vi "instr.UT61E.vi"(2 "error in (no error)":errorcluster caption="错误输入（无错误）", 3 "串口开关":bool, 4 "档位选择":enum16{"电流/mA", "电流/A", "电压/V"}(ring), 5 "VISA resource name":refnum<visa-resource-name> caption="VISA资源名称") -> (0 "error out":errorcluster caption="错误输出", 1 "结果":dbl)   [LabVIEW 2012, in "Lib_UEL.ATE.lvlib" / "Lib_Instrument.lvlib"]
uses:
  Lib_Instrument.lvlib
  <vilib>/Instr/_visa.llb/VISA Configure Serial Port (Instr).vi
panel:
  out "读取缓冲区":string
  # "1.电流电压均为直流测试时有效，且应打在对应的档位\n2.结果的单位与选择的单位一致\n                                             2013.6.18 Tina"
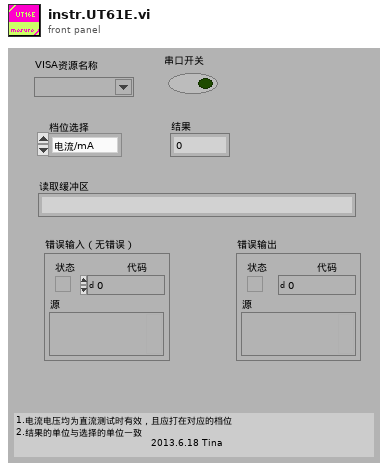
[diagram p1: front panel]
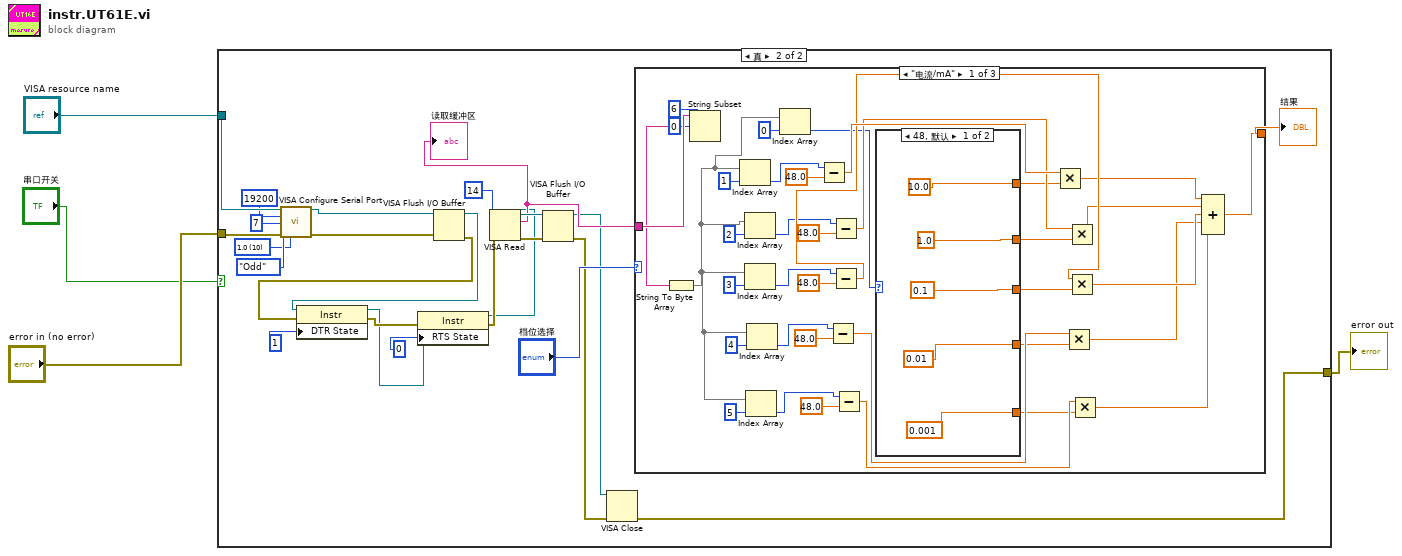
[diagram p0: block diagram]
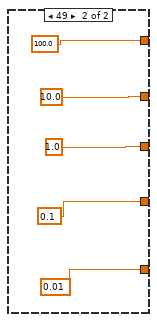
[diagram p3: hidden frame]
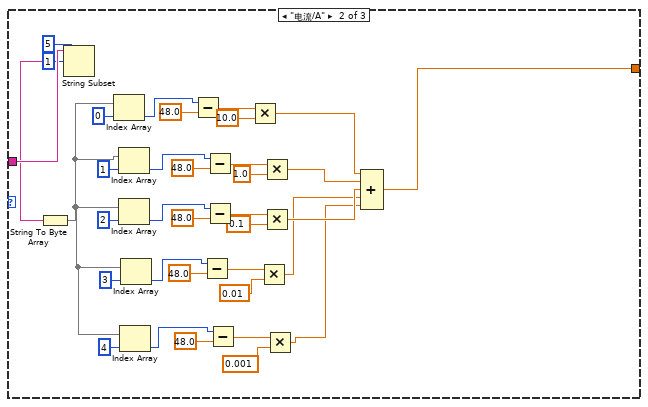
[diagram p4: hidden frame]
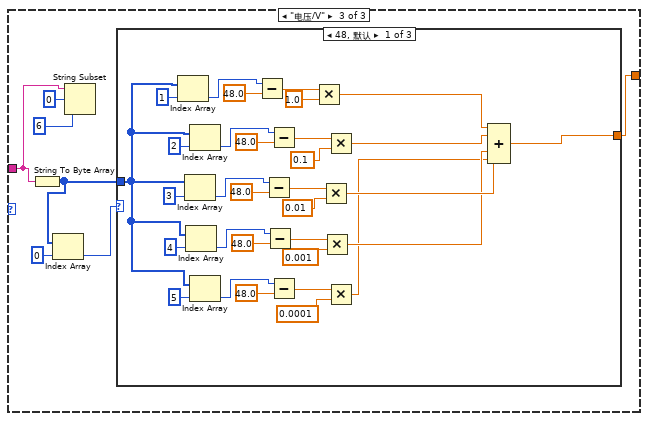
[diagram p5: hidden frame]
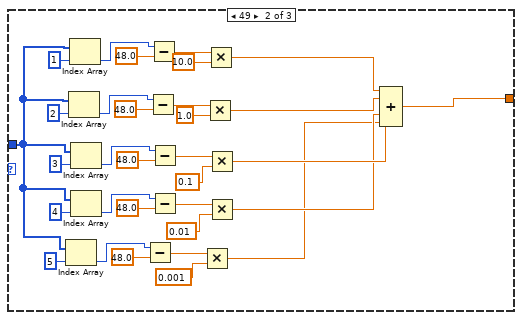
[diagram p6: hidden frame]
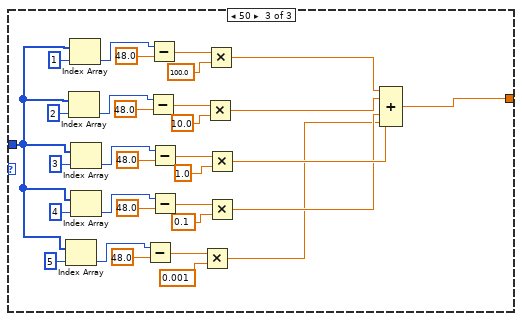
[diagram p7: hidden frame]
diagram:
  n1 = case shown="真" "串口开关" {
    tunnel: "VISA resource name" -> [_ w30]
    tunnel: "error in (no error)" -> [w5 w29]
    tunnel: [w5 w8] -> w1
    frame False {
    }
    frame True {
      w25 = u16 10 items=["1.0"=10, "1.5"=15, "2.0"=20] ("stop bits (10: 1 bit)")
      n2 = call-poly "VISA Configure Serial Port"("VISA resource name"=w30, "baud rate (9600)"=u32 19200, "data bits (8)"=u16 7, "parity (0:none)"=enum16{"None", "Odd", "Even", "Mark", "Space"}."Odd", "error in (no error)"=w29, "stop bits (10: 1 bit)"=w25) -> ("VISA resource name out"=w7:refnum<visa-resource-name>, "error out"=w6:errorcluster)  [unwired: 8 in]
      n3 = VISA Flush I/O Buffer(VISA resource name=w7, error in (no error)=w6) -> (VISA resource name out=w16:refnum<visa-resource-name>, error out=w15:errorcluster)  [unwired: 1 in]
      n4 = property class="Instr"(reference=w16, error in=w15, "DTR State"=1) -> (reference out=w13:refnum<visa-resource-name>, error out=w14:errorcluster)
      n5 = property class="Instr"(reference=w13, error in=w14, "RTS State"=0) -> (reference out=w11:refnum<visa-resource-name>, error out=w12:errorcluster)
      n6 = VISA Read(VISA resource name=w11, byte count=u32 14 ("字节总数"), error in (no error)=w12) -> (VISA resource name out=w23:refnum<visa-resource-name>, read buffer=w21:string, error out=w22:errorcluster)  [unwired: 1 out]
      "读取缓冲区" <- w21
      n7 = VISA Flush I/O Buffer(VISA resource name=w23, error in (no error)=w22) -> (VISA resource name out=w10:refnum<visa-resource-name>, error out=w9:errorcluster)  [unwired: 1 in]
      n8 = VISA Close(VISA resource name=w10, error in (no error)=w9) -> (error out=w8:errorcluster)
      n9 = case shown="\"电流/mA\"" "档位选择" {
        tunnel: w21 -> [w68 w114 w119]
        tunnel: [w34 w79 w115] -> w19
        frame "电流/mA" {
          n10 = String Subset(string=w68, offset (0)=0 ("偏移量(0)"), length (rest)=6 ("长度（剩余）")) -> (substring=w65:string)
          n11 = String To Byte Array(string=w65) -> (unsigned byte array=w32:u8[])
          n12 = Index Array(array=w32, index=1 ("索引")) -> (element=w45:u8)
          n13 = Index Array(array=w32, index=2 ("索引")) -> (element=w46:u8)
          n14 = Index Array(array=w32, index=3 ("索引")) -> (element=w47:u8)
          n15 = Index Array(array=w32, index=5 ("索引")) -> (element=w49:u8)
          n16 = Index Array(array=w32, index=4 ("索引")) -> (element=w48:u8)
          n17 = Index Array(array=w32, index=0 ("索引")) -> (element=w31:u8)
          n18 = Subtract(x=w45, y=48.0) -> (x-y=w58:dbl)
          n19 = Subtract(x=w48, y=48.0) -> (x-y=w52:dbl)
          n20 = Subtract(x=w46, y=48.0) -> (x-y=w57:dbl)
          n21 = Subtract(x=w47, y=48.0) -> (x-y=w55:dbl)
          n22 = Subtract(x=w49, y=48.0) -> (x-y=w51:dbl)
          n23 = case shown="48, 默认" w31 {
            tunnel: [10.0 ("y") 100.0 ("y")] -> w44
            tunnel: [1.0 ("y") 10.0 ("y")] -> w43
            tunnel: [0.1 ("y") 1.0 ("y")] -> w42
            tunnel: [0.01 ("y") 0.1 ("y")] -> w41
            tunnel: [0.001 ("y") 0.01 ("y")] -> w40
            frame 48, Default {
            }
            frame 49 {
            }
          }
          n24 = Multiply(x=w58, y=w44) -> (x*y=w39:dbl)
          n25 = Multiply(x=w52, y=w41) -> (x*y=w36:dbl)
          n26 = Multiply(x=w57, y=w43) -> (x*y=w38:dbl)
          n27 = Multiply(x=w55, y=w42) -> (x*y=w37:dbl)
          n28 = Multiply(x=w51, y=w40) -> (x*y=w35:dbl)
          n29 = Compound Arithmetic op=ADD(w39, w38, w37, w36, w35) -> (w34:dbl)
        }
        frame "电流/A" {
          n30 = String Subset(string=w114, offset (0)=1 ("偏移量(0)"), length (rest)=5 ("长度（剩余）")) -> (substring=w111:string)
          n31 = String To Byte Array(string=w111) -> (unsigned byte array=w110:u8[])
          n32 = Index Array(array=w110, index=0 ("索引")) -> (element=w90:u8)
          n33 = Index Array(array=w110, index=1 ("索引")) -> (element=w91:u8)
          n34 = Index Array(array=w110, index=2 ("索引")) -> (element=w92:u8)
          n35 = Index Array(array=w110, index=4 ("索引")) -> (element=w94:u8)
          n36 = Index Array(array=w110, index=3 ("索引")) -> (element=w93:u8)
          n37 = Subtract(x=w90, y=48.0) -> (x-y=w103:dbl)
          n38 = Subtract(x=w93, y=48.0) -> (x-y=w97:dbl)
          n39 = Subtract(x=w91, y=48.0) -> (x-y=w102:dbl)
          n40 = Subtract(x=w92, y=48.0) -> (x-y=w100:dbl)
          n41 = Subtract(x=w94, y=48.0) -> (x-y=w96:dbl)
          n42 = Multiply(x=w103, y=10.0) -> (x*y=w84:dbl)
          n43 = Multiply(x=w97, y=0.01) -> (x*y=w81:dbl)
          n44 = Multiply(x=w102, y=1.0) -> (x*y=w83:dbl)
          n45 = Multiply(x=w100, y=0.1) -> (x*y=w82:dbl)
          n46 = Multiply(x=w96, y=0.001) -> (x*y=w80:dbl)
          n47 = Compound Arithmetic op=ADD(w84, w83, w82, w81, w80) -> (w79:dbl)
        }
        frame "电压/V" {
          n48 = String To Byte Array(string=w119) -> (unsigned byte array=w116:u8[])
          n49 = Index Array(array=w116, index=0 ("索引")) -> (element=w117:u8)
          n50 = String Subset(string=w119, offset (0)=0 ("偏移量(0)"), length (rest)=6 ("长度（剩余）")) -> ()  [unwired: 1 out]
          n51 = case shown="48, 默认" w117 {
            tunnel: w116 -> [w124 w154 w186]
            tunnel: [w138 w170 w202] -> w115
            frame 48, Default {
              n52 = Index Array(array=w124, index=1 ("索引")) -> (element=w150:u8)
              n53 = Index Array(array=w124, index=3 ("索引")) -> (element=w142:u8)
              n54 = Index Array(array=w124, index=4 ("索引")) -> (element=w133:u8)
              n55 = Index Array(array=w124, index=2 ("索引")) -> (element=w149:u8)
              n56 = Index Array(array=w124, index=5 ("索引")) -> (element=w126:u8)
              n57 = Subtract(x=w150, y=48.0) -> (x-y=w151:dbl)
              n58 = Subtract(x=w142, y=48.0) -> (x-y=w143:dbl)
              n59 = Subtract(x=w133, y=48.0) -> (x-y=w132:dbl)
              n60 = Subtract(x=w149, y=48.0) -> (x-y=w148:dbl)
              n61 = Subtract(x=w126, y=48.0) -> (x-y=w127:dbl)
              n62 = Multiply(x=w151, y=1.0) -> (x*y=w141:dbl)
              n63 = Multiply(x=w143, y=0.01) -> (x*y=w139:dbl)
              n64 = Multiply(x=w132, y=0.001) -> (x*y=w123:dbl)
              n65 = Multiply(x=w148, y=0.1) -> (x*y=w140:dbl)
              n66 = Multiply(x=w127, y=0.0001) -> (x*y=w122:dbl)
              n67 = Compound Arithmetic op=ADD(w141, w140, w139, w123, w122) -> (w138:dbl)
            }
            frame 49 {
              n68 = Index Array(array=w154, index=5 ("索引")) -> (element=w158:u8)
              n69 = Index Array(array=w154, index=2 ("索引")) -> (element=w181:u8)
              n70 = Index Array(array=w154, index=1 ("索引")) -> (element=w182:u8)
              n71 = Index Array(array=w154, index=3 ("索引")) -> (element=w174:u8)
              n72 = Index Array(array=w154, index=4 ("索引")) -> (element=w165:u8)
              n73 = Subtract(x=w158, y=48.0) -> (x-y=w159:dbl)
              n74 = Subtract(x=w181, y=48.0) -> (x-y=w180:dbl)
              n75 = Subtract(x=w182, y=48.0) -> (x-y=w183:dbl)
              n76 = Subtract(x=w174, y=48.0) -> (x-y=w175:dbl)
              n77 = Subtract(x=w165, y=48.0) -> (x-y=w164:dbl)
              n78 = Multiply(x=w159, y=0.001) -> (x*y=w155:dbl)
              n79 = Multiply(x=w180, y=1.0) -> (x*y=w172:dbl)
              n80 = Multiply(x=w183, y=10.0) -> (x*y=w173:dbl)
              n81 = Multiply(x=w175, y=0.1) -> (x*y=w171:dbl)
              n82 = Multiply(x=w164, y=0.01) -> (x*y=w156:dbl)
              n83 = Compound Arithmetic op=ADD(w173, w172, w171, w156, w155) -> (w170:dbl)
            }
            frame 50 {
              n84 = Index Array(array=w186, index=5 ("索引")) -> (element=w190:u8)
              n85 = Index Array(array=w186, index=2 ("索引")) -> (element=w213:u8)
              n86 = Index Array(array=w186, index=1 ("索引")) -> (element=w214:u8)
              n87 = Index Array(array=w186, index=3 ("索引")) -> (element=w206:u8)
              n88 = Index Array(array=w186, index=4 ("索引")) -> (element=w197:u8)
              n89 = Subtract(x=w190, y=48.0) -> (x-y=w191:dbl)
              n90 = Subtract(x=w213, y=48.0) -> (x-y=w212:dbl)
              n91 = Subtract(x=w214, y=48.0) -> (x-y=w215:dbl)
              n92 = Subtract(x=w206, y=48.0) -> (x-y=w207:dbl)
              n93 = Subtract(x=w197, y=48.0) -> (x-y=w196:dbl)
              n94 = Multiply(x=w191, y=0.001) -> (x*y=w187:dbl)
              n95 = Multiply(x=w212, y=10.0) -> (x*y=w204:dbl)
              n96 = Multiply(x=w215, y=100.0) -> (x*y=w205:dbl)
              n97 = Multiply(x=w207, y=1.0) -> (x*y=w203:dbl)
              n98 = Multiply(x=w196, y=0.1) -> (x*y=w188:dbl)
              n99 = Compound Arithmetic op=ADD(w205, w204, w203, w188, w187) -> (w202:dbl)
            }
          }
        }
      }
      "结果" <- w19
    }
  }
  "error out" <- w1
